vi "Set Output Impedance.vi"(8 "error in (no error)":errorcluster, 9 "User Define Impedance":dbl=50.0 caption="User-Defined Impedance (50 Ohms)" min=1.0 max=10000.0 format="%.2f", 10 "Impedance":u16(ring) caption="Impedance (0: 50 Ohms)" items=["50 Ohms", "High Impedance", "User Defined"], 11 "Agilent 33210A in":refnum<class "Agilent 33210A.lvclass">) -> (0 "error out":errorcluster, 3 "Agilent 33210A out":refnum<class "Agilent 33210A.lvclass">)   [LabVIEW 2021, in "Func Generator.lvlib" / "Agilent 33210A.lvclass"]
uses:
  Agilent 33210A.lvclass
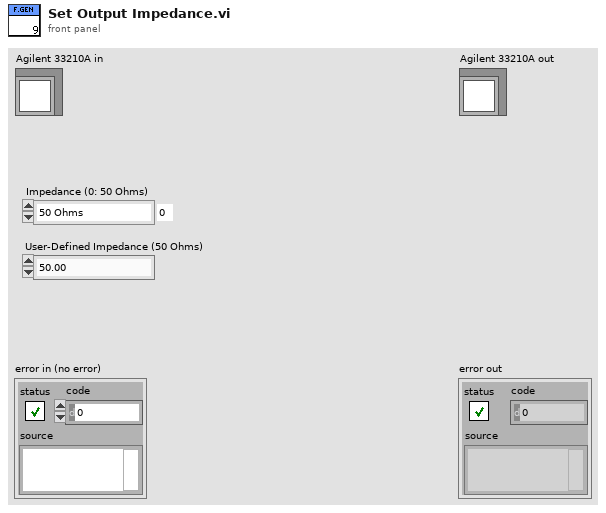
[diagram p1: front panel]
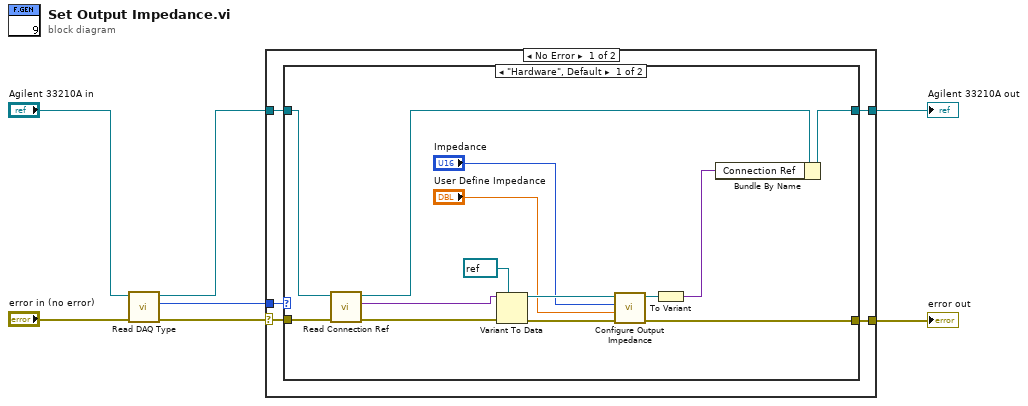
[diagram p0: block diagram]
diagram:
  n1 = call-dynamic "Read DAQ Type.vi"("error in (no error)"="error in (no error)", "Agilent 33210A in"="Agilent 33210A in") -> ("error out"=w6:errorcluster, "DAQ Type"=w5:enum16{"Hardware", "Simulation"}, "Agilent 33210A out"=w1:refnum<class "Agilent 33210A.lvclass">)  [unwired: 7 in]
  n2 = case shown="No Error" w6 {
    selector: w6 -> [w11 w29]
    tunnel: w5 -> [w12 _]
    tunnel: w1 -> [w10 w30]
    tunnel: [w9 w30] -> w3
    tunnel: [w8 w29] -> w2
    frame No Error {
      n3 = case shown="\"Hardware\", Default" w12 {
        tunnel: w11 -> [w26 w27]
        tunnel: w10 -> [w14 w28]
        tunnel: [w17 w28] -> w9
        tunnel: [w18 w27] -> w8
        frame "Hardware", Default {
          n4 = call-dynamic "Read Connection Ref.vi"("error in (no error)"=w26, "Agilent 33210A in"=w14) -> ("error out"=w25:errorcluster, "Connection Ref"=w24:variant, "Agilent 33210A out"=w13:refnum<class "Agilent 33210A.lvclass">)  [unwired: 7 in]
          n5 = Variant To Data(error in=w25, type=refnum<visa-resource-name> refnum ("VISA resource name"), Variant=w24) -> (data=w21:refnum<visa-resource-name>, error out=w22:errorcluster)
          n6 = call <instrlib>:"Configure Output Impedance.vi"("error in (no error)"=w22, "User-Defined Impedance (50 Ohms)"="User Define Impedance", "Impedance (0: 50 Ohms)"="Impedance", "VISA resource name"=w21) -> ("error out"=w18:errorcluster, "VISA resource name out"=w16:refnum<visa-resource-name>)  [unwired: 6 in]
          n7 = To Variant(anything=w16) -> (Variant=w15:variant)
          n8 = Bundle By Name(cluster=w13, "Connection Ref"=w15) -> (w17:refnum<class "Agilent 33210A.lvclass">)
        }
        frame "Simulation" {
        }
      }
    }
    frame Error {
    }
  }
  "error out" <- w2
  "Agilent 33210A out" <- w3
